vi "getRobotPose.vi"(8 "error in":errorcluster) -> (0 "error out":errorcluster, 3 "Pose":T1 format="%.3f")   [LabVIEW 2013]
uses:
  <vilib>/Analysis/Matrix/Datatypes/RealMatrix.ctl
  ROS/Code/SubVIs/BaxterSide.ctl
  ROS/Code/Console/Servers/ServerSubs/(nist) Arm Globals.vi
  NIST2/Prim/Fwd Kenimatics - array.vi
  <vilib>/Analysis/Matrix/NI_Matrix.lvlib
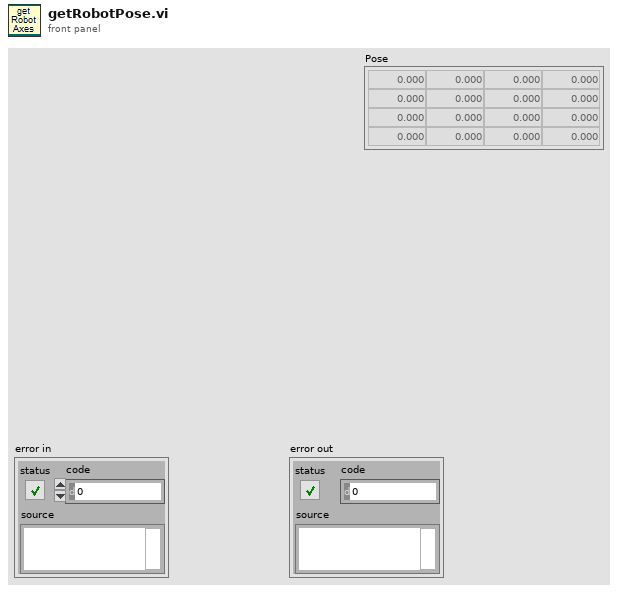
[diagram p1: front panel]
types:
  T1 = typedef "NI_Matrix.lvlib/RealMatrix.ctl" = dbl[][]
  T2 = typedef "BaxterSide.ctl" = enum16{"left", "right"}
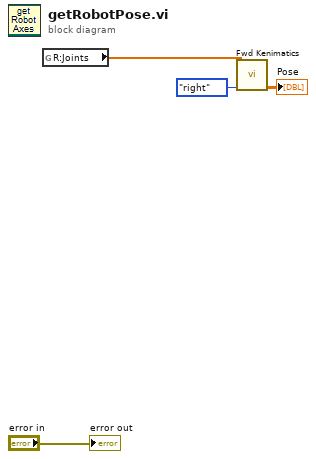
[diagram p0: block diagram]
diagram:
  n1 = global read "(nist) Arm Globals.vi" "R:Joints"() -> (w2:dbl[])
  n2 = call-poly "Fwd Kenimatics.vi"("Side"=BaxterSide."right", "Joints"=w2) -> ("Matrix"=→"Pose":T1)  [unwired: 8 in, 1 out]
  "error out" <- "error in"
